vi "addCommandToQueue.vi"(8 "error in (no error)":errorcluster, 10 "Command.lvclass":refnum<class "Command.lvclass">, 11 "Monochromator in":refnum<class "Monochromator.lvclass">) -> (0 "error out":errorcluster, 3 "Monochromator out":refnum<class "Monochromator.lvclass">)   [LabVIEW 2016, in "Monochromator.lvclass"]
uses:
  Monochromator.lvclass
  Commands/Command/Command.lvclass
  Monochromator.lvclass/Monochromator.ctl
  Commands/Command/Command.lvclass/Command.ctl
  Commands/CommandQueue/CommandQueue.lvclass
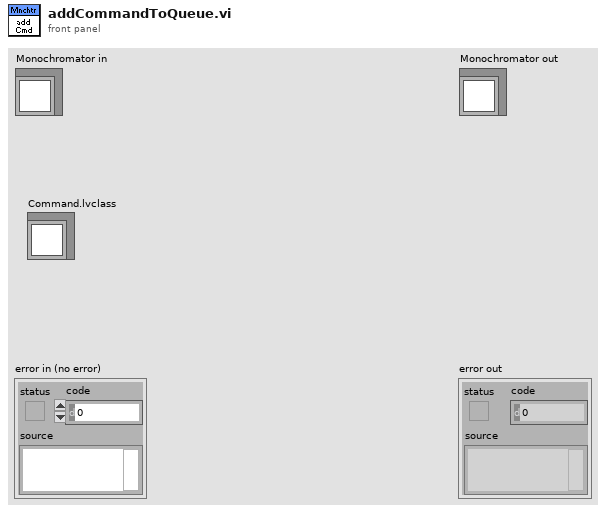
[diagram p1: front panel]
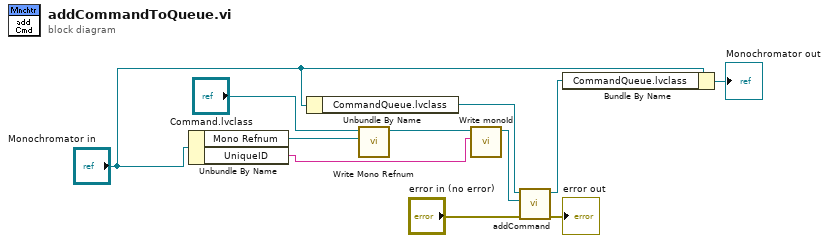
[diagram p0: block diagram]
diagram:
  n1 = Unbundle By Name("Monochromator in") -> ("Mono Refnum"=w3:refnum<k7>, "UniqueID"=w4:string)
  n2 = Unbundle By Name("Monochromator in") -> ("CommandQueue.lvclass"=w10:refnum<class "CommandQueue.lvclass">)
  n3 = call "Write Mono Refnum.vi"("Mono Refnum"=w3, "Command in"="Command.lvclass") -> ("Command out"=w5:refnum<class "Command.lvclass">)  [unwired: 8 in, 1 out]
  n4 = call "Write monoId.vi"("monoId"=w4, "Command in"=w5) -> ("Command out"=w1:refnum<class "Command.lvclass">)  [unwired: 8 in, 1 out]
  n5 = call "addCommand.vi"("error in (no error)"="error in (no error)", "Command.lvclass"=w1, "CommandQueue in"=w10) -> ("error out"=→"error out":errorcluster, "CommandQueue out"=w9:refnum<class "CommandQueue.lvclass">)  [unwired: 7 in]
  n6 = Bundle By Name(cluster="Monochromator in", "CommandQueue.lvclass"=w9) -> (→"Monochromator out":refnum<class "Monochromator.lvclass">)
